vi "driveStraight.vi"(6 "Use Camera":bool, 8 "Reset Encoders":bool, 9 "Do Speed Control?":bool, 10 "Speed (ft/sec)":dbl, 11 "Distance":dbl) -> ()   [LabVIEW 2011]
uses:
  signals/Signal.ctl
  drivetrain/gear_shift_state.ctl
  drivetrain/drivetrain_drive_mode.ctl
  drivetrain/drivetrain_drive_write_thread.ctl
  Auto_Conf.vi
  drivetrain/drivetrain_globals.vi
panel:
  in  "cam lim":dbl
  in  "Integral Cap":dbl
  in  "cam gain":dbl=0.5
  out "Distance (in)":cluster{"Left":dbl, "Right":dbl}
  in  "drift gain":dbl=-1.25
  in  "low speed const":dbl=3.3
  in  "drive gain":dbl=0.04
  out "Initial Error":dbl
  out "Waveform Chart":dbl(graph)
  in  "Bias":cluster{"Left":dbl, "Right":dbl}={"Left"=1.0, "Right"=0.95}
  in  "Max Delta Per Iteration":dbl=0.15
  in  "Overshoot":dbl=18.0
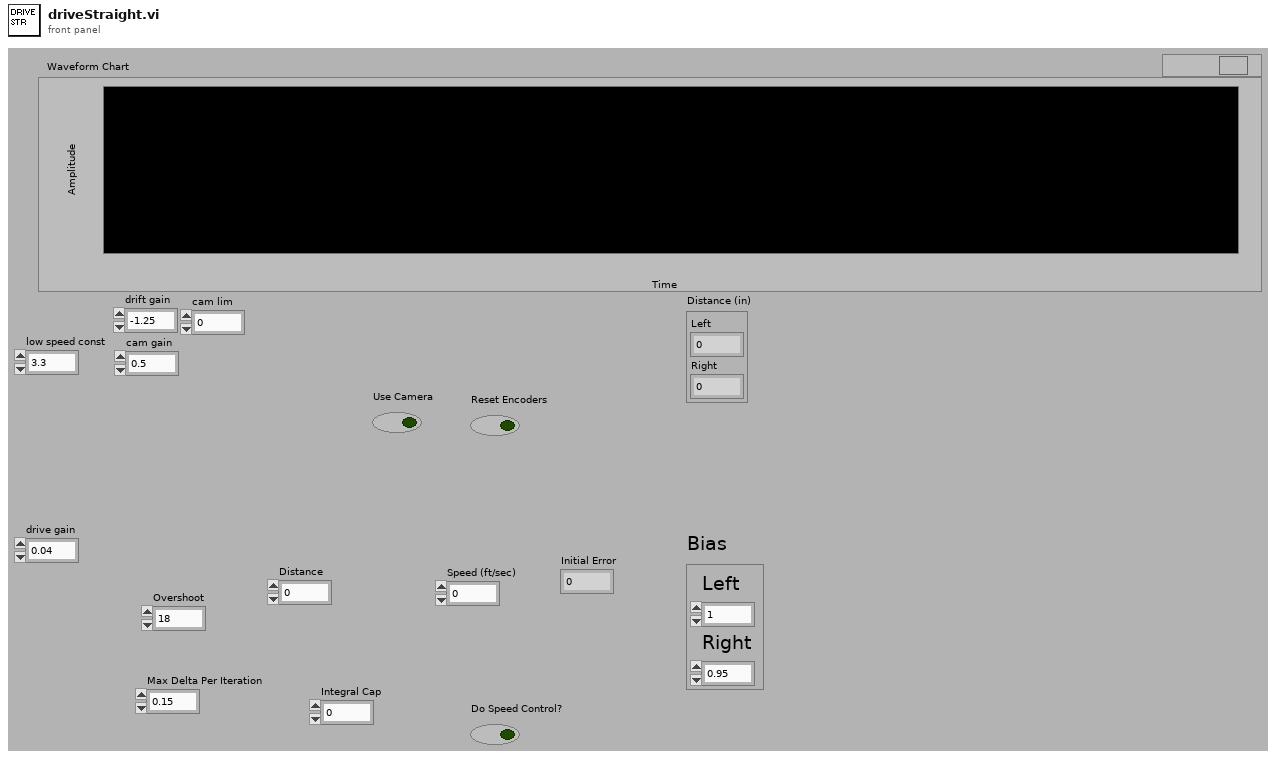
[diagram p1: front panel]
types:
  T1 = typedef "WPI_GyroDevRef.ctl" = cluster{"DevStatus":errorcluster, "Analog Module":T2, "Analog Channel":T3, "Offset":dbl, "Gain (VoltsPerDegree/Second)":dbl}
  T2 = typedef "FPGA_TypedefAnalogModule.ctl" = enum16{"Analog Module 1", "Analog Module 2"}
  T3 = typedef "FPGA_AIChannel.ctl" = enum8{"AI 1", "AI 2", "AI 3", "AI 4", "AI 5", "AI 6", "AI 7", "AI 8", "Invalid"}
  T4 = typedef "Signal.ctl" = enum16{"SIGFIRE", "SIGSTOPSCRIPT", "SIGSTARTGUN", "SIGSTOPGUN", "SIGDISABLED", "SIGENABLED", "SIGUDPTIMEOUT", "SIGNEWVISION_REMOTE", "SIGNEWVISION_LOCAL", "SIGSHOTFIRED", "SIGDOTRACK", "SIGDONTTRACK"}
  T5 = typedef "gear_shift_state.ctl" = enum16{"low", "high"}
  T6 = typedef "drivetrain_drive_mode.ctl" = enum16{"open loop", "closed loop"}
  T7 = enum16{"Get Latest Data", "Get Local Data", "Get Remote Data", "Set Local Data", "Set Remote Data"}
  T8 = typedef "drivetrain_drive_write_thread.ctl" = enum16{"Teleop", "Script Engine - Autonomous", "Script Engine - Sequence"}
  T9 = typedef "Camera State.ctl" = enum16{"No Targets", "Low Confidence", "Medium Confidence", "High Confidence", "Camera Error"}
  T10 = cluster{"X Position":dbl, "Distance":dbl, "Camera State":T9}
  T11 = typedef "WPI_RobotDriveDevRef.ctl" = cluster{"DevStatus":errorcluster, "Motors[]":T12[], "Square Inputs":bool, "Max Output":dbl}
  T12 = typedef "WPI_MotorControlDeviceRef.ctl" = cluster{"DeviceStatus":errorcluster, "Type":enum16{"PWM", "CAN"}, "PWM":cluster{"Digital Module":T13, "PWM Channel":T14, "DeadBand":T15}, "CAN":cluster{"Device Number":u8, "Control Mode":T16, "Semaphore":T17, "Max Vout":dbl}, "Invert":bool, "TransformRef":T18, "InvTransformRef":T18}
  T13 = typedef "FPGA_TypedefDigitalModule.ctl" = enum16{"Digital Module 1", "Digital Module 2"}
  T14 = typedef "FPGA_DIOPWMChannel.ctl" = enum8{"PWM 1", "PWM 2", "PWM 3", "PWM 4", "PWM 5", "PWM 6", "PWM 7", "PWM 8", "PWM 9", "PWM 10", "Invalid"}
  T15 = typedef "WPI_PWMDeadband.ctl" = cluster{"Name":string, "maxPositivePwm":i32, "minPositivePwm":i32, "centerPwm":i32, "maxNegativePwm":i32, "minNegativePwm":i32, "angularRange":u16}
  T16 = typedef "WPI_CANJaguar_ControlMode.ctl" = enum8{"Percent VBus", "Current", "Speed", "Position", "Voltage"}
  T17 = typedef "Semaphore RefNum" = refnum<k1>
  T18 = typedef "WPI_PWMTransform_ConPane.ctl" = refnum<vi>
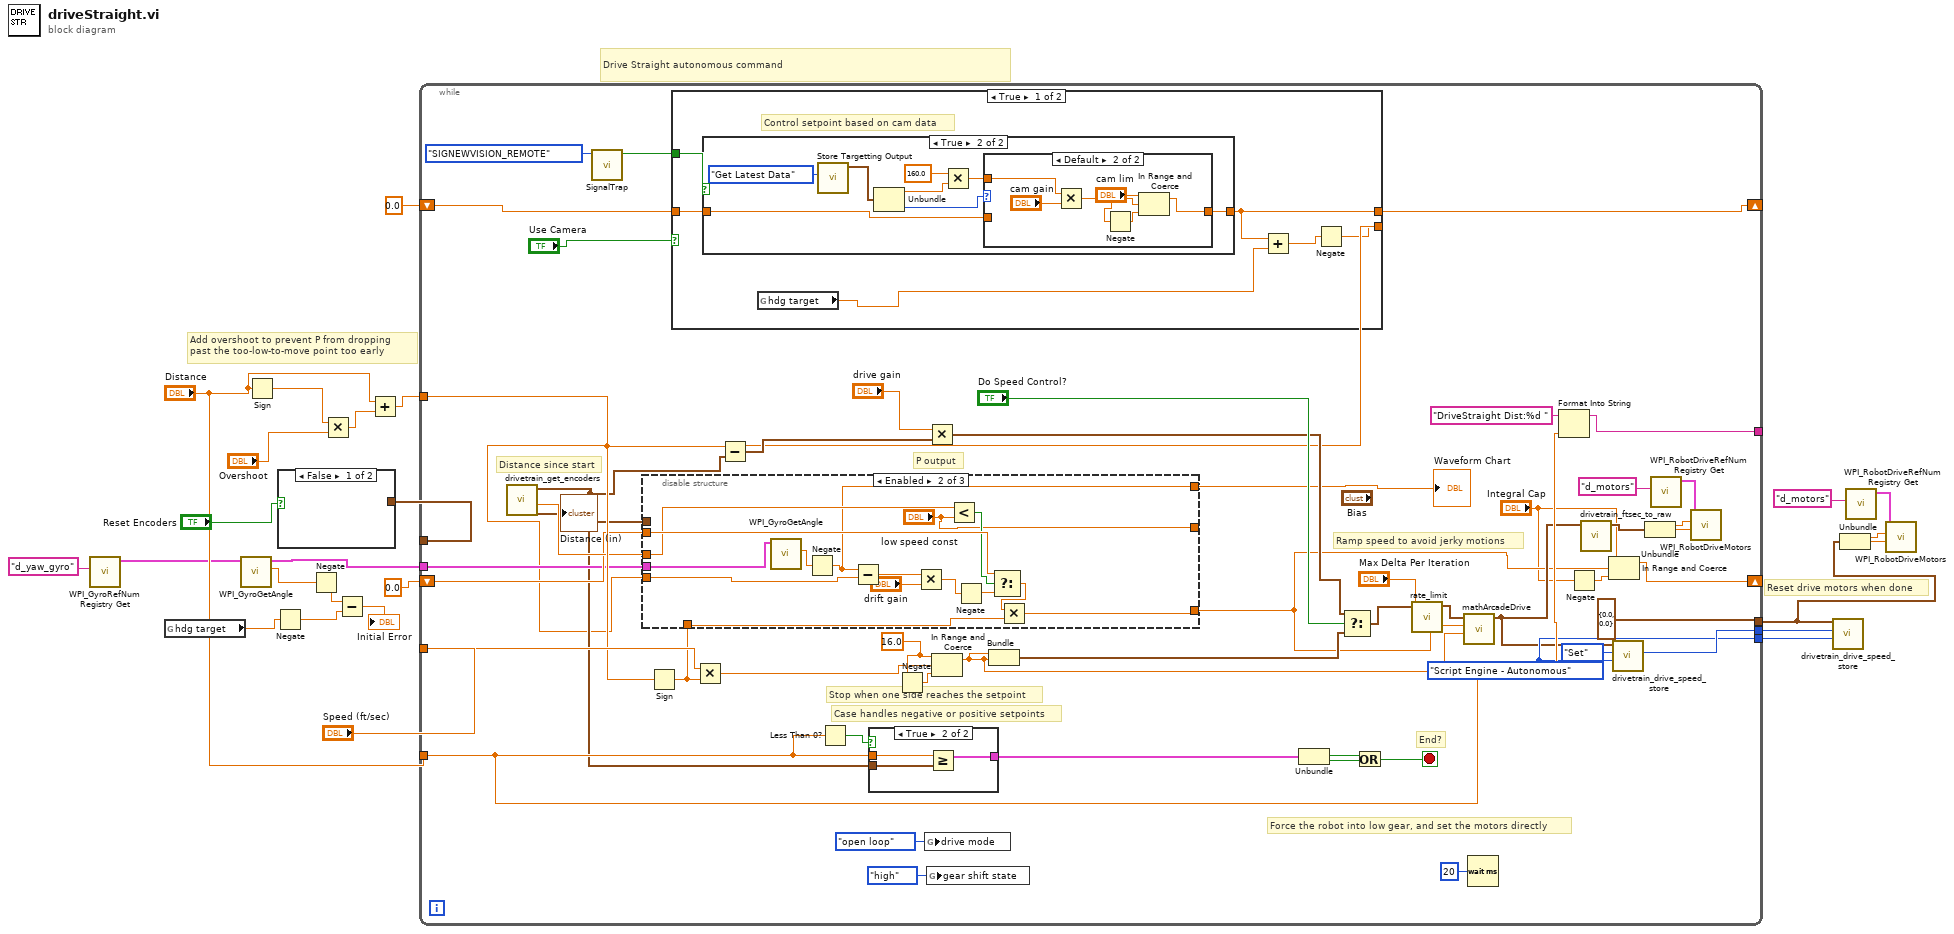
[diagram p0: block diagram]
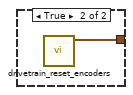
[diagram p2: hidden frame]
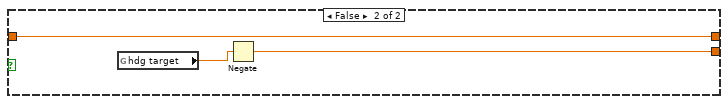
[diagram p5: hidden frame]
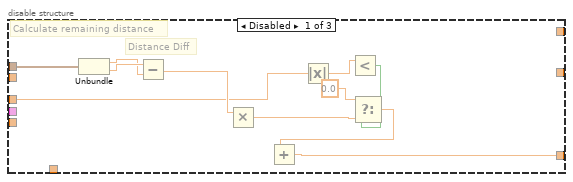
[diagram p6: hidden frame]
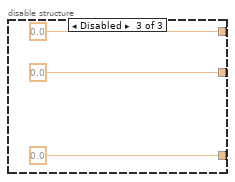
[diagram p7: hidden frame]
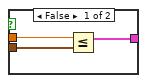
[diagram p8: hidden frame]
diagram:
  # "Drive Straight autonomous command"
  # "Reset drive motors when done"
  # "Add overshoot to prevent P from dropping\npast the too-low-to-move point too early"
  n1 = call <vilib>:"WPI_GyroRefNum Registry Get.vi"("refnum name"="d_yaw_gyro") -> ("GyroDevRef"=w5:T1)  [unwired: 1 in, 9 out]
  n2 = global read "Auto_Conf.vi" "hdg target"() -> (w4:dbl)
  n3 = call <vilib>:"WPI_GyroGetAngle.vi"("GyroDevRef"=w5) -> ("Angle"=w12:dbl)  [unwired: 1 in, 9 out]
  n4 = Sign(1:"Distance") -> (0:w19:dbl)
  n5 = Negate(x=w4) -> (-x=w3:dbl)
  n6 = case shown="False" "Reset Encoders" {
    tunnel: [_ w25] -> w23
    frame False {
    }
    frame True {
      n7 = call "drivetrain_reset_encoders.vi"() -> ("Distance (in)"=w25:cluster{"Left":dbl, "Right":dbl})  [unwired: 9 in, 2 out]
    }
  }
  n8 = Negate(x=w12) -> (-x=w11:dbl)
  n9 = Multiply(x=w19, y="Overshoot") -> (x*y=w21:dbl)
  n10 = Subtract(x=w11, y=w3) -> (x-y=→"Initial Error":dbl)
  n11 = Add(x="Distance", y=w21) -> (x+y=w22:dbl)
  n12 = while {
    tunnel: "Speed (ft/sec)" -> [w58]
    tunnel: w23 -> [_]
    tunnel: w22 -> [w56]
    tunnel: [cluster{"Left":dbl, "Right":dbl} {"Left"=0.0, "Right"=0.0} ("Drive")] -> w8
    tunnel: "Distance" -> [w63]
    tunnel: [w62] -> _
    shift-right: [w28] -> _
    shift-left: 0.0 -> [w50]
    tunnel: w5 -> [w48]
    tunnel: [w46] -> w14
    tunnel: [w45] -> w13
    shift-right: [w32] -> _
    shift-left: 0.0 -> [w33]
    stop <- w72 stop-if-true
    w45 = drivetrain_drive_write_thread."Script Engine - Autonomous" ("Write Thread")
    w46 = enum16{"Set", "Get"}."Set" ("data_store_mode")
    w65 = 16.0
    # "Case handles negative or positive setpoints"
    # "End?"
    # "Ramp speed to avoid jerky motions"
    # "P output"
    # "Force the robot into low gear, and set the motors directly"
    # "Stop when one side reaches the setpoint"
    # "Distance since start"
    n13 = call "drivetrain_get_encoders.vi"() -> ("Avg Velocity (Ft/Sec)"=w55:dbl, "Distance (in)"=w43:cluster{"Left":dbl, "Right":dbl})  [unwired: 9 in, 1 out]
    "Distance (in)" <- w43
    n14 = call "SignalTrap.vi"("Signal"=Signal."SIGNEWVISION_REMOTE") -> ("Trapped Signal"=w30:bool)  [unwired: 10 in]
    n15 = Sign(1:w56) -> (0:w49:dbl)
    n16 = case shown="True" "Use Camera" {
      tunnel: [w77 w99] -> w35
      tunnel: w33 -> [w80 w98]
      tunnel: [w79 w98] -> w32
      tunnel: w30 -> [w81 _]
      frame True {
        # "Control setpoint based on cam data"
        n17 = case shown="True" w81 {
          tunnel: [w82 w85] -> w79
          tunnel: w80 -> [w82 w86]
          frame False {
          }
          frame True {
            n18 = call "Store Targetting Output.vi"("mode"=T7."Get Latest Data") -> ("Targetting Output"=w89:T10)  [unwired: 10 in]
            n19 = Unbundle(w89) -> ("X Position"=w88:dbl, "Camera State"=w84:T9)  [unwired: 1 out]
            n20 = Multiply(x=160.0, y=w88) -> (x*y=w83:dbl)
            n21 = case shown="Default" w84 {
              tunnel: w86 -> [w91 _]
              tunnel: [w91 w94] -> w85
              tunnel: w83 -> [_ w97]
              frame "No Targets" {
              }
              frame Default {
                n22 = Multiply(x=w97, y="cam gain") -> (x*y=w95:dbl)
                n23 = Negate(x="cam lim") -> (-x=w93:dbl)
                n24 = In Range and Coerce(upper limit="cam lim", x=w95, lower limit=w93) -> (coerced(x)=w94:dbl)  [unwired: 1 out]
              }
            }
          }
        }
        n25 = global read "Auto_Conf.vi" "hdg target"() -> (w76:dbl)
        n26 = Add(x=w79, y=w76) -> (x+y=w78:dbl)
        n27 = Negate(x=w78) -> (-x=w77:dbl)
      }
      frame False {
        n28 = global read "Auto_Conf.vi" "hdg target"() -> (w100:dbl)
        n29 = Negate(x=w100) -> (-x=w99:dbl)
      }
    }
    n30 = disable-structure shown="Enabled" {
      disable-tunnel: [w105 w121 0.0 ("Wheel")] -> w29
      disable-tunnel: w43 -> [w104 _ _]
      disable-tunnel: w55 -> [w103 w125 _]
      disable-tunnel: [_ w116 0.0 ("Waveform Chart")] -> w51
      disable-tunnel: w50 -> [_ w126 _]
      disable-tunnel: [_ "low speed const" 0.0 ("low speed const")] -> _
      disable-tunnel: w49 -> [_ w120 _]
      disable-tunnel: w48 -> [_ w119 _]
      disable-tunnel: w35 -> [_ w118 _]
      frame Disabled {
        # "Distance Diff"
        # "Calculate remaining distance"
        n31 = Unbundle(w104) -> ("Left"=w111:dbl, "Right"=w112:dbl)
        n32 = Subtract(x=w112, y=w111) -> (x-y=w114:dbl)
        n33 = Multiply(x=w114) -> (y=w113:dbl, x*y=w102:dbl)
        n34 = Absolute Value(x=w103) -> (abs(x)=w109:dbl)
        n35 = Less?(x=w109) -> (y=w108:dbl, x < y?=w107:bool)
        n36 = Select(t=0.0, s=w107, f=w102) -> (s? t:f=w101:dbl)
        n37 = Add(x=w101) -> (y=w110:dbl, x+y=w105:dbl)
      }
      frame Enabled {
        n38 = call <vilib>:"WPI_GyroGetAngle.vi"("GyroDevRef"=w119) -> ("Angle"=w115:dbl)  [unwired: 1 in, 9 out]
        n39 = Negate(x=w115) -> (-x=w116:dbl)
        n40 = Subtract(x=w116, y=w118) -> (x-y=w117:dbl)
        n41 = Multiply(x=w117, y="drift gain") -> (x*y=w128:dbl)
        n42 = Less?(x=w125, y="low speed const") -> (x < y?=w124:bool)
        n43 = Negate(x=w128) -> (-x=w127:dbl)
        n44 = Select(t=w126, s=w124, f=w127) -> (s? t:f=w122:dbl)
        n45 = Multiply(x=w122, y=w120) -> (x*y=w121:dbl)
      }
      frame Disabled {
      }
    }
    "Waveform Chart" <- w51
    n46 = Multiply(x=w58, y=w49) -> (x*y=w57:dbl)
    n47 = Subtract(x=w56, y=w43) -> (x-y=w69:cluster{"Left":dbl, "Right":dbl})
    n48 = Less Than 0?(x=w63) -> (x < 0?=w68:bool)
    n49 = case shown="True" w68 {
      tunnel: w63 -> [w135 w138]
      tunnel: w43 -> [w134 w137]
      tunnel: [w133 w136] -> w75
      frame False {
        n50 = Less Or Equal?(x=w135, y=w134) -> (x <= y?=w133:cluster{"Left":bool, "Right":bool})
      }
      frame True {
        n51 = Greater Or Equal?(x=w138, y=w137) -> (x >= y?=w136:cluster{"Left":bool, "Right":bool})
      }
    }
    n52 = Negate(x=w65) -> (-x=w66:dbl)
    n53 = global write "drivetrain_globals.vi" "drive mode"(drivetrain_drive_mode."open loop" ("drive mode")) -> ()
    n54 = Multiply(x="drive gain", y=w69) -> (x*y=w54:cluster{"Left":dbl, "Right":dbl})
    n55 = global write "drivetrain_globals.vi" "gear shift state"(gear_shift_state."high" ("gear shift state")) -> ()
    n56 = In Range and Coerce(upper limit=w65, x=w57, lower limit=w66) -> (coerced(x)=w60:dbl)  [unwired: 1 out]
    n57 = Bundle(w60, w60) -> (w59:cluster{dbl, dbl})  [unwired: 1 out]
    n58 = Unbundle(w75) -> ("Left"=w74:bool, "Right"=w73:bool)
    n59 = Select(t=w54, s="Do Speed Control?", f=w59) -> (s? t:f=w53:cluster{"Left":dbl, "Right":dbl})
    n60 = Or(x=w74, y=w73) -> (x .or. y?=w72:bool)
    n61 = call "rate_limit.vi"("Max Delta Per Iteration"="Max Delta Per Iteration", "Drive"=w53) -> ("Output"=w52:cluster{"Left":dbl, "Right":dbl})  [unwired: 9 in]
    n62 = call "mathArcadeDrive.vi"("Range"=w60, "Wheel"=w29, "Throttle"=w52) -> ("Drive"=w36:cluster{"Left":dbl, "Right":dbl})  [unwired: 8 in]
    n63 = Wait (ms)(milliseconds to wait=u32 20) -> ()  [unwired: 1 out]
    n64 = Format Into String(initial string="DriveStraight Dist:%d ", w63) -> (resulting string=w62:string)  [unwired: 2 in, 1 out]
    n65 = Negate(x="Integral Cap") -> (-x=w27:dbl)
    n66 = call "drivetrain_ftsec_to_raw.vi"("Drive Data"=w36) -> ("Drive Data Out"=w37:cluster{"Left":dbl, "Right":dbl})  [unwired: 10 in]
    n67 = In Range and Coerce(upper limit="Integral Cap", x=w29, lower limit=w27) -> (coerced(x)=w28:dbl)  [unwired: 1 out]
    n68 = call "drivetrain_drive_speed_store.vi"("Write Thread"=w45, "data_store_mode"=w46, "drive data"=w36) -> ()  [unwired: 7 in, 2 out]
    n69 = Unbundle(w37) -> ("Left"=w39:dbl, "Right"=w40:dbl)
    n70 = call <vilib>:"WPI_RobotDriveRefNum Registry Get.vi"("refnum name"="d_motors") -> ("RobotDriveDevRef"=w42:T11)  [unwired: 9 in, 1 out]
    n71 = call <vilib>:"WPI_RobotDriveMotors.vi"("RightSpeed"=w40, "LeftSpeed"=w39, "RobotDriveDevRef"=w42) -> ()  [unwired: 7 in, 2 out]
  }
  n72 = call "drivetrain_drive_speed_store.vi"("Write Thread"=w13, "data_store_mode"=w14, "drive data"=w8) -> ()  [unwired: 7 in, 2 out]
  n73 = Unbundle(w8) -> ("Left"=w10:dbl, "Right"=w9:dbl)
  n74 = call <vilib>:"WPI_RobotDriveRefNum Registry Get.vi"("refnum name"="d_motors") -> ("RobotDriveDevRef"=w6:T11)  [unwired: 9 in, 1 out]
  n75 = call <vilib>:"WPI_RobotDriveMotors.vi"("RightSpeed"=w9, "LeftSpeed"=w10, "RobotDriveDevRef"=w6) -> ()  [unwired: 7 in, 2 out]
